vi "SongTimer.vi"(6 "Time":dbl, 8 "error in (no error)":errorcluster, 9 "Mode":T1=enum."Play", 10 "Message Queues in":T2, 11 "UI Refs in":T3) -> (0 "error out":errorcluster, 3 "UI Refs out":T3)   [LabVIEW 2015]
uses:
  Controls & Type Defs/UI Data.ctl
  support/Message Queue/All Message Queues.ctl
  support/Message Queue/Message Cluster.ctl
  Controls & Type Defs/SongTimerModes.ctl
  support/Message Queue/Enqueue Message (Single).vi
  support/Message Queue/Message Queue.lvlib
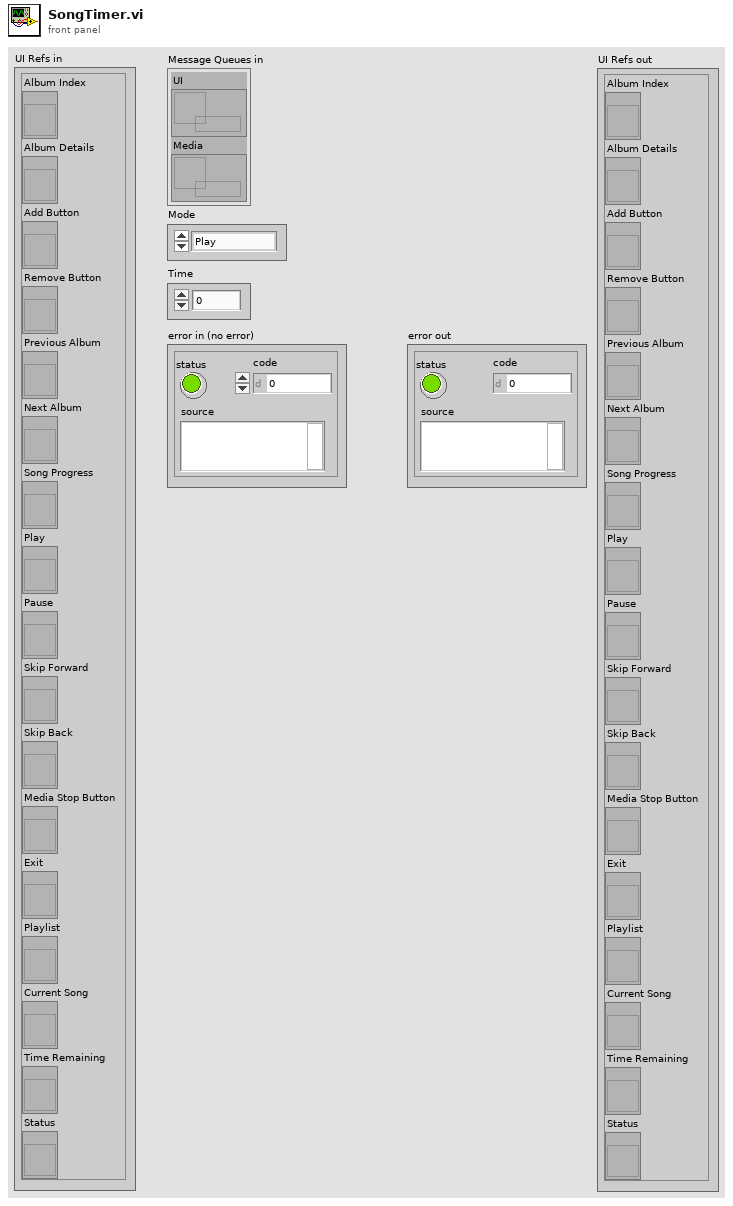
[diagram p1: front panel]
types:
  T1 = typedef "SongTimerModes.ctl" = enum16{"Start", "Play", "Jump"}
  T2 = typedef "Message Queue.lvlib/All Message Queues.ctl" = cluster{"UI":refnum<queue>, "Media":refnum<queue>}
  T3 = typedef "UI Data.ctl" = cluster{"Album Index":refnum<vi>, "Album Details":refnum<vi>, "Add Button":refnum<vi>, "Remove Button":refnum<vi>, "Previous Album":refnum<vi>, "Next Album":refnum<vi>, "Song Progress":refnum<vi>, "Play":refnum<vi>, "Pause ":refnum<vi>, "Skip Forward":refnum<vi>, "Skip Back":refnum<vi>, "Media Stop Button":refnum<vi>, "Exit":refnum<vi>, "Playlist":refnum<vi>, "Current Song":refnum<vi>, "Time Remaining":refnum<vi>, "Status":refnum<vi>}
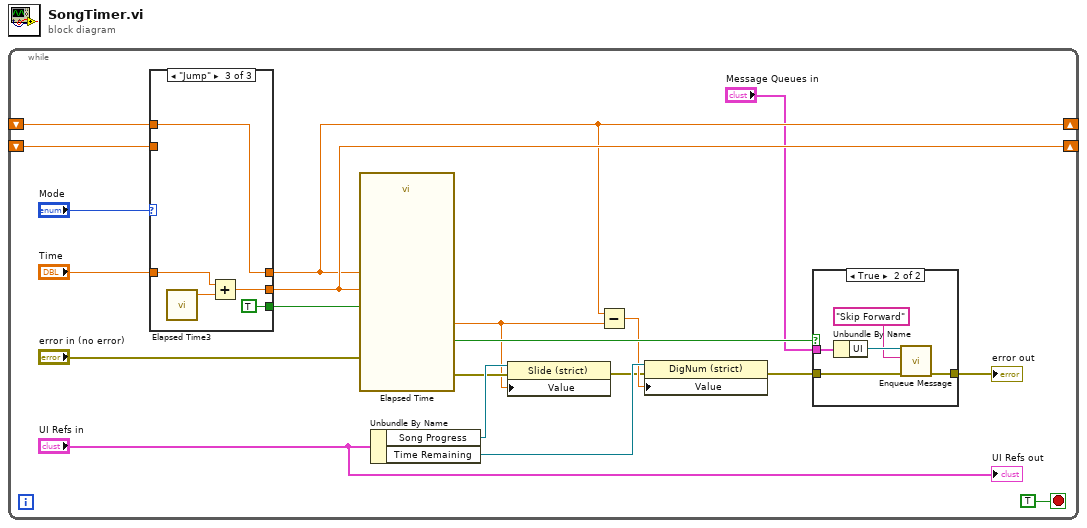
[diagram p0: block diagram]
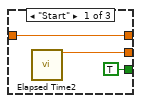
[diagram p3: hidden frame]
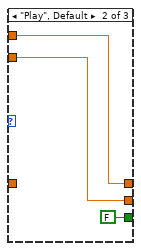
[diagram p4: hidden frame]
diagram:
  n1 = while {
    shift-right: [w8] -> _
    shift-left: _ -> [w16]
    shift-right: [w15] -> _
    shift-left: _ -> [w14]
    stop <- TRUE stop-if-true
    n2 = case shown="\"Jump\"" "Mode" {
      tunnel: [w29 w32 w37] -> w8
      tunnel: "Time" -> [w29 _ w34]
      tunnel: w16 -> [_ w32 w37]
      tunnel: [w27 w31 w33] -> w15
      tunnel: w14 -> [_ w31 _]
      tunnel: [TRUE ("Reset") FALSE ("Reset") TRUE ("Reset")] -> w12
      frame "Start" {
        n3 = call "Elapsed Time2"() -> ("Present (s)"=w27:dbl)  [unwired: 12 in, 7 out]
      }
      frame "Play", Default {
      }
      frame "Jump" {
        n4 = call "Elapsed Time3"() -> ("Present (s)"=w35:dbl)  [unwired: 12 in, 7 out]
        n5 = Add(x=w34, y=w35) -> (x+y=w33:dbl)
      }
    }
    n6 = call "Elapsed Time"("Time Target (s)"=w8, "Reset"=w12, "error in (no error)"="error in (no error)", "Set Start Time (s)"=w15) -> ("Elapsed Time (s)"=w1:dbl, "Time has Elapsed"=w20:bool, "error out"=w10:errorcluster)  [unwired: 8 in, 5 out]
    n7 = Unbundle By Name("UI Refs in") -> ("Song Progress"=w11:refnum<vi>, "Time Remaining"=w9:refnum<vi>)
    n8 = property class="Slide (strict)"(reference=w11, error in=w10, "Value"=w1) -> (error out=w6:errorcluster)  [unwired: 1 out]
    n9 = Subtract(x=w8, y=w1) -> (x-y=w7:dbl)
    n10 = property class="DigNum (strict)"(reference=w9, error in=w6, "Value"=w7) -> (error out=w5:errorcluster)  [unwired: 1 out]
    n11 = case shown="True" w20 {
      tunnel: w5 -> [w21 w26]
      tunnel: [w21 w25] -> w4
      tunnel: "Message Queues in" -> [_ w24]
      frame False {
      }
      frame True {
        n12 = Unbundle By Name(w24) -> ("UI"=w23:refnum<queue>)
        n13 = call-poly "Enqueue Message.vi"("error in (no error)"=w26, "Message"="Skip Forward", "Message Queue"=w23) -> ("error out"=w25:errorcluster)  [unwired: 7 in, 1 out]
      }
    }
    "error out" <- w4
    "UI Refs out" <- "UI Refs in"
  }
